vi "get_path_git.vi"(8 "error in (no error)":errorcluster) -> (0 "error out":errorcluster, 3 "git.exe":path)   [LabVIEW 2015, in "lv-bin-git.lvlib"]
uses:
  lv-bin-git.lvlib
  <userlib>/antonio-alexander/lv-bin/lv-bin/public/api/v1/v1.lvlib
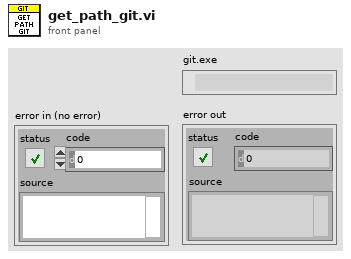
[diagram p1: front panel]
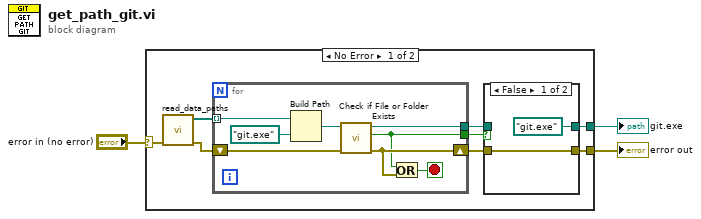
[diagram p0: block diagram]
diagram:
  n1 = case shown="No Error" "error in (no error)" {
    selector: "error in (no error)" -> [w11 w24]
    tunnel: [w4 w24] -> w3
    tunnel: [w6 _] -> w1
    frame No Error {
      n2 = call <userlib>:"read_data_paths.vi"("error in (no error)"=w11) -> ("error out"=w10:errorcluster, "path [] out"=w9:path[])  [unwired: 9 in]
      n3 = for {
        tunnel: w9 -> [w17] mode=indexing
        shift-right: [w16] -> w5
        shift-left: w10 -> [w19]
        tunnel: [w18] -> w8
        tunnel: [w14] -> w7
        stop <- w15 stop-if-true
        n4 = Build Path(base path=w17, name or relative path=path "git.exe" ("Application Directory")) -> (appended path=w13:path)
        n5 = call <vilib>:"Check if File or Folder Exists.vi"("error in (no error)"=w19, "path"=w13) -> ("error out"=w16:errorcluster, "file or folder exists?"=w14:bool, "dup path"=w18:path)  [unwired: 7 in]
        n6 = Or(x=w14, y=w16) -> (x .or. y?=w15:bool)
      }
      n7 = case shown="False" w7 {
        tunnel: w8 -> [_ w23]
        tunnel: [path "git.exe" ("dup path") w23] -> w6
        tunnel: w5 -> [w21 w22]
        tunnel: [w21 w22] -> w4
        frame False {
        }
        frame True {
        }
      }
    }
    frame Error {
    }
  }
  "error out" <- w3
  "git.exe" <- w1
